vi "MoveRelative.vi"(8 "Error In":errorcluster, 10 "Move Relative Value":dbl, 11 "Thorlabs In":refnum<class "Thorlabs.lvclass">) -> (0 "Error Out":errorcluster, 3 "Thorlabs Out":refnum<class "Thorlabs.lvclass">)   [LabVIEW 2018, in "Thorlabs.lvlib" / "Thorlabs.lvclass"]
doc: "Moves the Axis by a relative distance from its current location.\n\nCreator: Slade Jeppesen\nCreated Date: 09/29/20"
uses:
  Thorlabs.lvclass
  Thorlabs.lvclass/Thorlabs.ctl
  C:/AME Test Engineering/LabVIEW/PPLs/Axis/DLLs/ThorLabs.MotionControl.KCube.DCServoCLI.dll
  PPLs/Axis/DLLs/ThorLabs.MotionControl.KCube.DCServoCLI.dll
  6a7749ec-2137-4f45-b8f1-2887bde184ae.vi
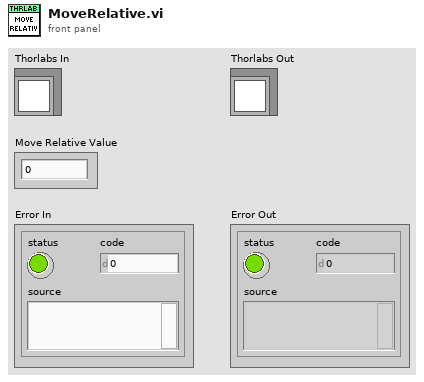
[diagram p1: front panel]
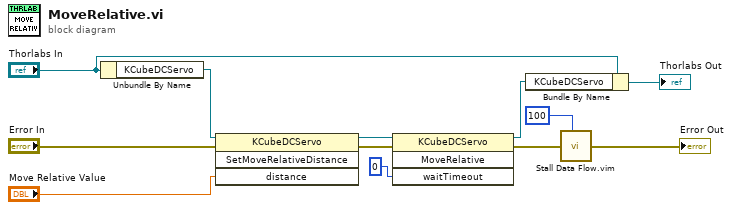
[diagram p0: block diagram]
diagram:
  n1 = Unbundle By Name("Thorlabs In") -> ("KCubeDCServo"=w12:refnum<k24>)
  n2 = invoke class="KCubeDCServo" method="SetMoveRelativeDistance"(reference=w12, error in="Error In", "distance"="Move Relative Value") -> (reference out=w10:refnum<k24>, error out=w11:errorcluster)  [unwired: 1 in, 2 out]
  n3 = invoke class="KCubeDCServo" method="MoveRelative"(reference=w10, error in=w11, "waitTimeout"=0) -> (reference out=w9:refnum<k24>, error out=w3:errorcluster)  [unwired: 1 in, 2 out]
  n4 = Bundle By Name(cluster="Thorlabs In", "KCubeDCServo"=w9) -> (→"Thorlabs Out":refnum<class "Thorlabs.lvclass">)
  n5 = call "Stall Data Flow.vim"("value in"=w3, "milliseconds to wait"=u32 100) -> ("value out"=→"Error Out":errorcluster)  [unwired: 1 out]
